vi "Excel_OpenReference_v2.vi"(5 "Template File Path":string="C:\\Users\\Candan\\Documents\\Sales Documents\\Gebze Customers\\Tubitak\\UME\\Guc Lab\\Ozlem Yilmaz\\TestStand Projesi\\14 Agustos 2015\\LVFiles\\Support\\Format_Table.xltx", 8 "error in (no error)":errorcluster, 11 "Excel._Application":refnum<k7>) -> (0 "error out":errorcluster, 1 "Sheets Reference Out":refnum<k7>, 2 "Workbook Reference Out":refnum<k7>, 3 "Excel Application Reference Out":refnum<k7>)   [LabVIEW 2014]
doc: "This VI demonstrates the use of ActiveX to write a table into a Microsoft Excel worksheet."
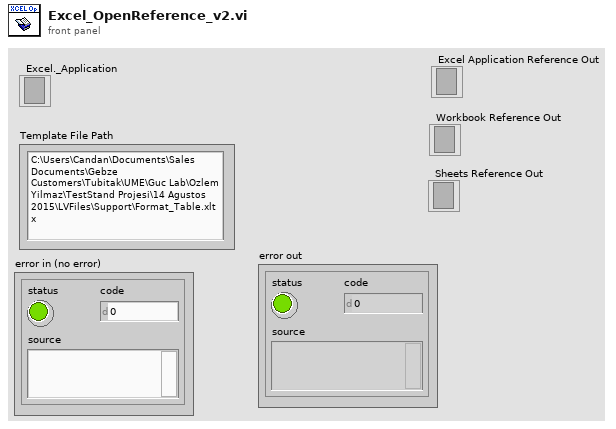
[diagram p1: front panel]
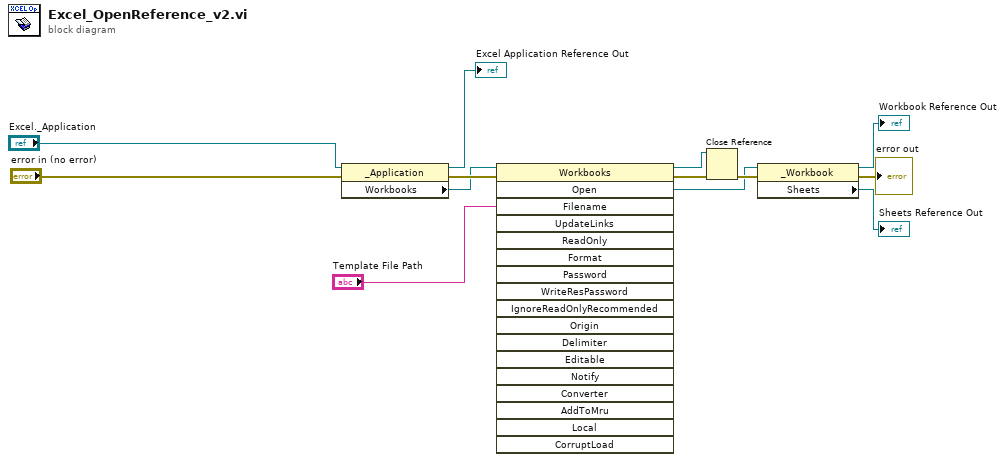
[diagram p0: block diagram]
diagram:
  n1 = property class="_Application"(reference="Excel._Application", error in="error in (no error)") -> (reference out=→"Excel Application Reference Out":refnum<k7>, error out=w13:errorcluster, "Workbooks"=w9:refnum<k7>)
  n2 = invoke class="Workbooks" method="Open"(reference=w9, error in=w13, "Filename"="Template File Path") -> (reference out=w11:refnum<k7>, error out=w12:errorcluster, "Open"=w8:refnum<k7>)  [unwired: 15 in, 15 out]
  n3 = Close Reference(reference=w11, error in (no error)=w12) -> (error out=w10:errorcluster)
  n4 = property class="_Workbook"(reference=w8, error in=w10) -> (reference out=→"Workbook Reference Out":refnum<k7>, error out=→"error out":errorcluster, "Sheets"=→"Sheets Reference Out":refnum<k7>)
